vi "Stop Core.vi"(10 "final error code":i32, 11 "Car Wash Model in":refnum<class "Car Wash Model.lvclass">) -> (3 "Car Wash Model out":refnum<class "Car Wash Model.lvclass">)   [LabVIEW 2019, in "Car Wash Model.lvclass"]
doc: "(<B>Filename</B>: Actor Framework.lvlib:Actor.lvclass:Stop Core.vi)\n\nDefines what the actor does before it stops. Use the <B>final error code</B> input to determine whether the actor shut down in response to an error.\n\nBy default, this method does nothing. A descendant class may override it to define behavior, such as shutting down any processes the actor initiated in its override of the Actor Core method."
uses:
  <vilib>/gpm_packages/@cs/Car-wash/Source/Car Wash Model/Car Wash Model/Car Wash Model.lvclass
  <vilib>/gpm_packages/@cs/Car-wash/Source/Car Wash Model/Car Wash Model/Car Wash Model.lvclass/Car Wash Model.ctl
  <vilib>/gpm_packages/@cs/mva-core/Source/IModel/IModel/IModel.lvclass
  <vilib>/gpm_packages/@cs/Car-wash/Source/Fan Controller Ref/Fan Controller Ref.lvclass
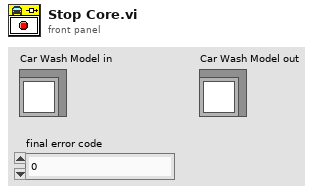
[diagram p1: front panel]
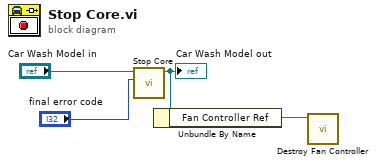
[diagram p0: block diagram]
diagram:
  n1 = call-parent "Stop Core.vi"("final error code"="final error code", "IObserver in"="Car Wash Model in") -> ("IObserver out"=w2:refnum<class "Car Wash Model.lvclass">)  [unwired: 9 in]
  "Car Wash Model out" <- w2
  n2 = Unbundle By Name(w2) -> ("Fan Controller Ref"=w1:refnum<data-value>)
  n3 = call <vilib>:"Destroy Fan Controller.vi"("Fan Controller Ref"=w1) -> ()  [unwired: 10 in, 1 out]
